vi "1DInt16ArrayToNode(viaString).vi"(0 "Tree DVR in":refnum<data-value>, 1 "I16 array in":i16[](array[numeric]), 3 "error in (no error)":errorcluster, 4 "NodePath":string) -> (7 "error out":errorcluster)   [LabVIEW 2014]
uses:
  <vilib>/MDSplus/Classes/Tree_Class/Tree.lvclass
  <vilib>/MDSplus/Library/MDSplus.lvlib
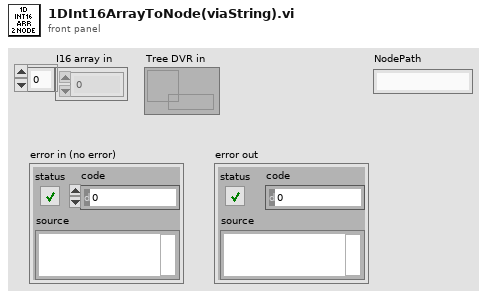
[diagram p1: front panel]
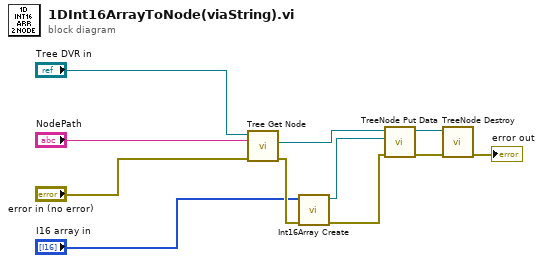
[diagram p0: block diagram]
diagram:
  n1 = call <vilib>:"Tree Get Node.vi"("error in (no error)"="error in (no error)", "Path"="NodePath", "Tree DVR in"="Tree DVR in") -> ("error out"=w8:errorcluster, "Node out"=w6:refnum<data-value>)  [unwired: 6 in, 1 out]
  n2 = call <vilib>:"Int16Array Create.vi"("error in (no error)"=w8, "I16 array in"="I16 array in") -> ("error out"=w7:errorcluster, "Int16Array DVR out"=w5:refnum<data-value>)  [unwired: 8 in]
  n3 = call <vilib>:"TreeNode Put Data.vi"("error in (no error)"=w7, "Data"=w5, "TreeNode DVR in"=w6) -> ("error out"=w4:errorcluster, "TreeNode DVR out"=w3:refnum<data-value>)  [unwired: 7 in]
  n4 = call <vilib>:"TreeNode Destroy.vi"("error in (no error)"=w4, "TreeNode DVR in"=w3) -> ("error out"=→"error out":errorcluster)  [unwired: 9 in]
